vi "PicoScope5000aAWG.vi"(6 "Arbitrary Waveform Settings":T2 {"Index Mode" items=["Single", "Dual", "Quad"]}, 7 "Standard Waveform Settings":T1={"Start Frequency"=1000.0, "Stop Frequency"=1000.0, "Increment"=0.0, "Dwell Time (seconds)"=0.0} {"Stop Frequency" min=0.03 max=1000000.0; "Start Frequency" min=0.03 max=1000000.0}, 9 "General AWG Settings":T3={"Peak-to-Peak Voltage (microvolts)"=2000000, "Offset Voltage (microvolts)"=0, "Wave Type"=0, "Sweep Type"=0, "Shots"=0, "Sweeps"=0, "Trigger Type"=0, "Trigger Source"=0, "Ext. Threshold (ADC count)"=0, "White Noise/PRBS"=0} {"White Noise/PRBS" items=["Normal", "White Noise", "PRBS"]; "Trigger Source" items=["None", "Scope Trigger", "Aux. In", "Ext. In", "Software Trigger"]; "Trigger Type" items=["Rising", "Falling", "Gate High", "Gate Low"]; "Sweep Type" items=["Up", "Down", "Up-Down", "Down-Up"]; "Wave Type" items=["Sine", "Square", "Triangle", "Ramp Up", "Ramp Down", "Sinc", "Gaussian", "Half Sine", "DC", "Arbitrary"]}, 10 "Handle In":i16, 11 "error in":errorcluster) -> (0 "Trigger Source Out":u32, 1 "Arbitrary\nWaveform Graph":i16[](graph), 2 "Handle Out":i16, 3 "error out":errorcluster)   [LabVIEW 2010]
doc: "This VI can be used to control the arbitrary waveform generator. Standard waveforms can be selected or arbitrary waveform can be selected under 'Wave Type'. There are three settings clusters: general settings that apply to both arbitrary and standard waveforms, settings that apply only to standard waveforms and settings that apply only to arbitrary waveforms. It is not necessary to connect all of these clusters if only using arbitrary waveforms or only using standard waveforms are required.\n\nWhen selecting arbitrary waveform, it is necessary to specify a text file containing the wave form. This text file should have a single value on each line in the range -1 to 1. For further information on the settings, see descriptions of ps3000aSetSigGenBuiltIn and ps3000aSetSigGenArbitrary."
uses:
  ps5000a.dll
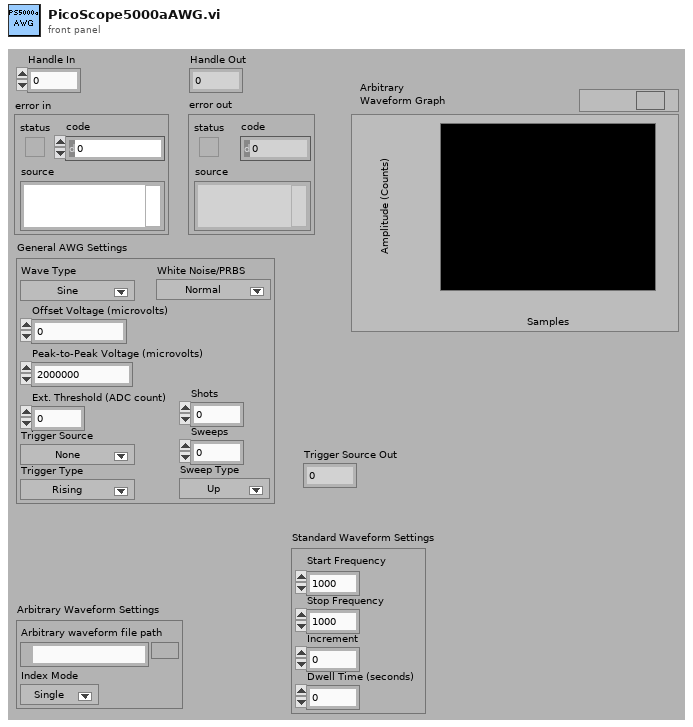
[diagram p1: front panel]
types:
  T1 = cluster{"Start Frequency":dbl, "Stop Frequency":dbl, "Increment":dbl, "Dwell Time (seconds)":dbl}
  T2 = cluster{"Arbirary waveform file path":path, "Index Mode":u32}
  T3 = cluster{"Peak-to-Peak Voltage (microvolts)":u32, "Offset Voltage (microvolts)":i32, "Wave Type":u32, "Sweep Type":u32, "Shots":u32, "Sweeps":u32, "Trigger Type":u32, "Trigger Source":u32, "Ext. Threshold (ADC count)":i16, "White Noise/PRBS":u32}
  T4 = cluster{"status":bool, "code":u32, "source":string}
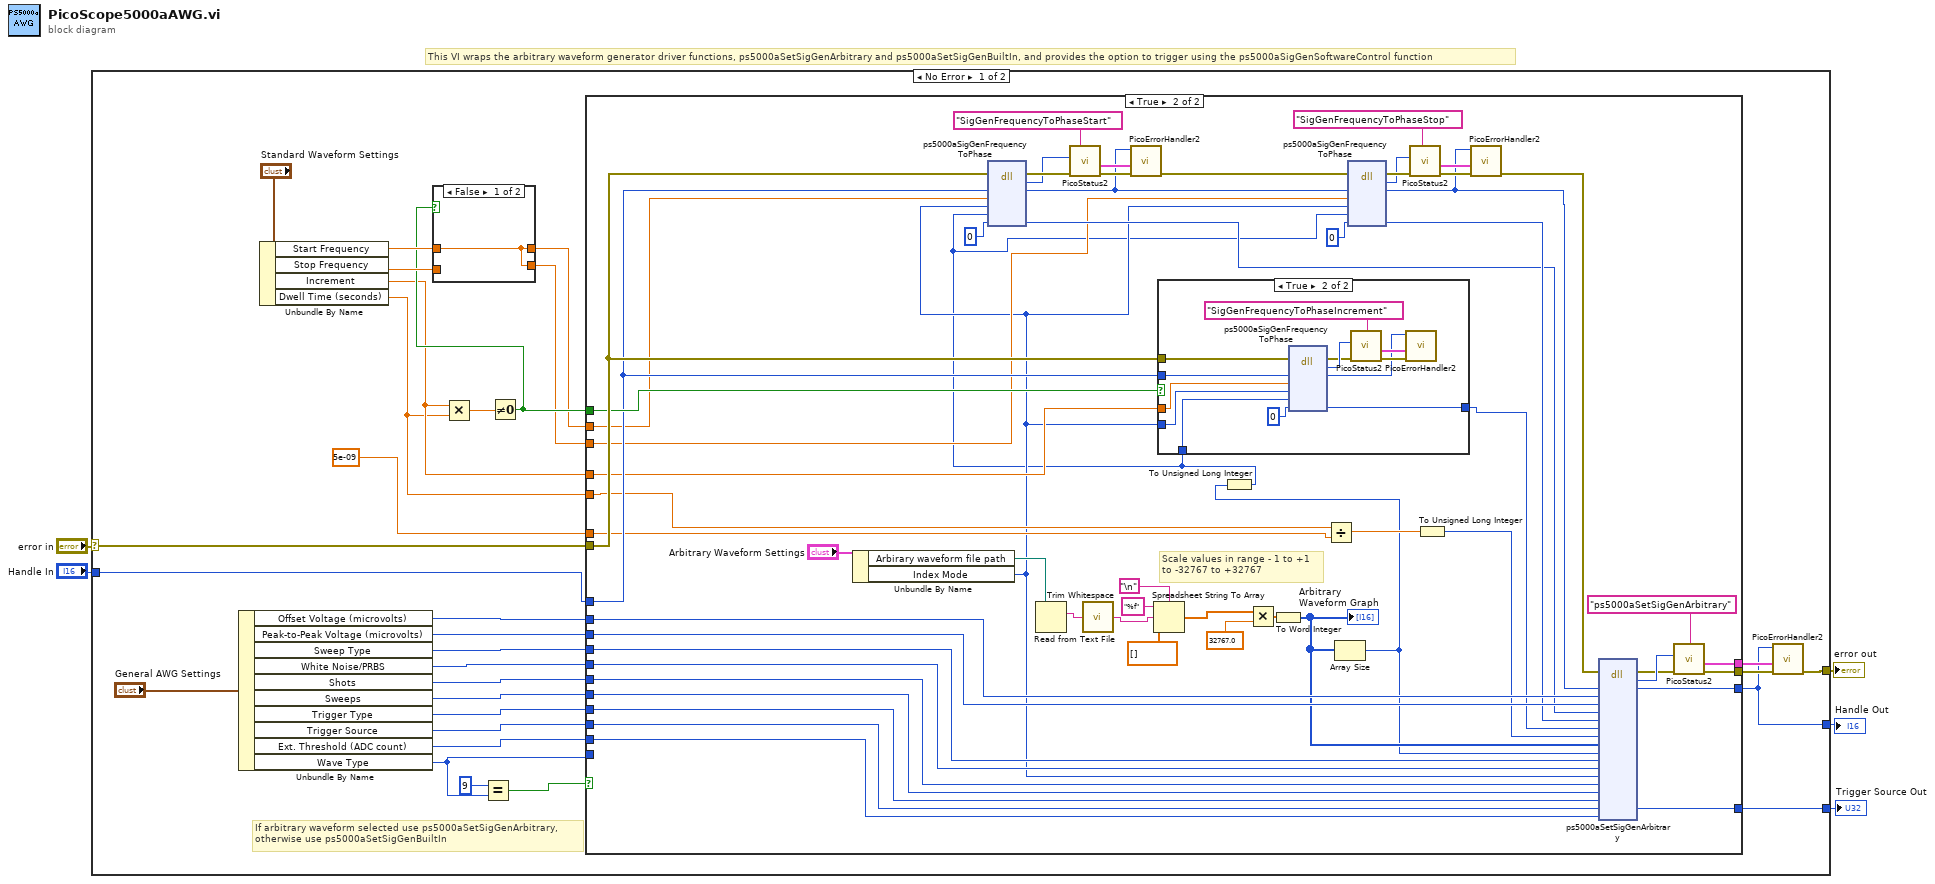
[diagram p0: block diagram]
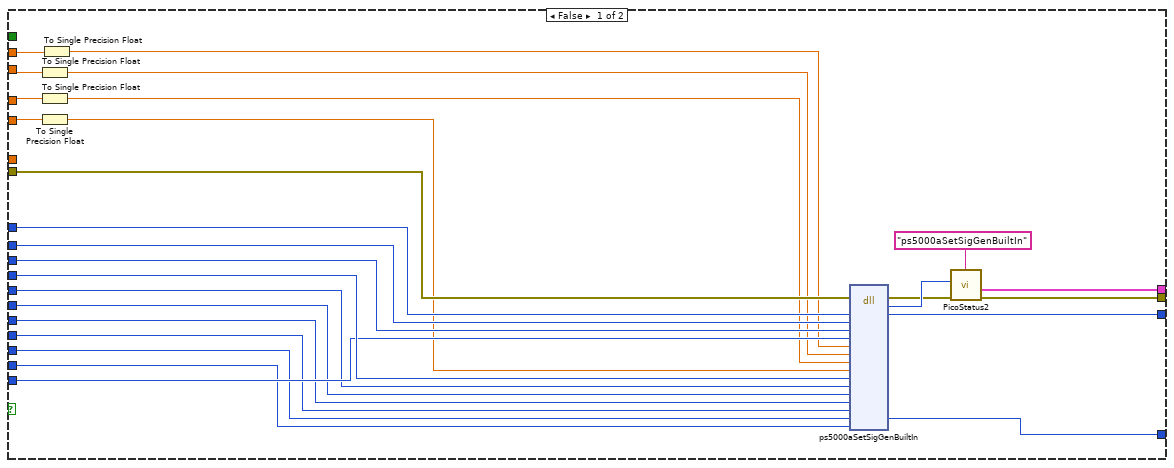
[diagram p3: hidden frame]
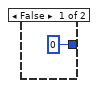
[diagram p4: hidden frame]
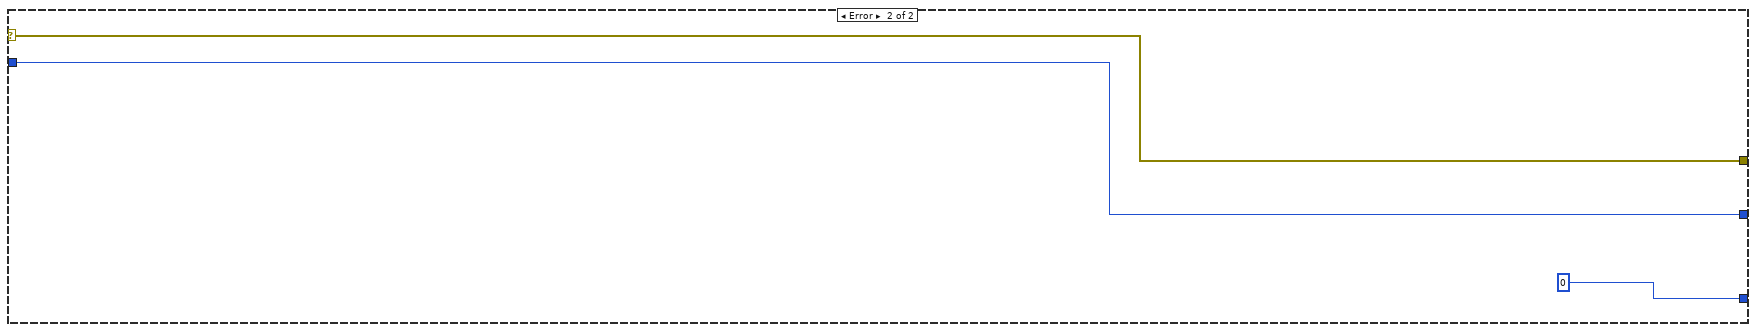
[diagram p5: hidden frame]
diagram:
  # "This VI wraps the arbitrary waveform generator driver functions, ps5000aSetSigGenArbitrary and ps5000aSetSigGenBuiltIn, and provides the option to trigger using the ps5000aSigGenSoftwareControl function"
  n1 = case shown="No Error" "error in" {
    selector: "error in" -> [w20 w141]
    tunnel: [w6 w140] -> w5
    tunnel: "Handle In" -> [w33 w140]
    tunnel: [w32 w141] -> w3
    tunnel: [w18 0] -> w1
    frame No Error {
      # "If arbitrary waveform selected use ps5000aSetSigGenArbitrary, \notherwise use ps5000aSetSigGenBuiltIn"
      n2 = Unbundle By Name("General AWG Settings") -> ("Offset Voltage (microvolts)"=w30:i32, "Peak-to-Peak Voltage (microvolts)"=w29:u32, "Sweep Type"=w28:u32, "White Noise/PRBS"=w27:u32, "Shots"=w26:u32, "Sweeps"=w25:u32, "Trigger Type"=w24:u32, "Trigger Source"=w23:u32, "Ext. Threshold (ADC count)"=w22:i16, "Wave Type"=w21:u32)
      n3 = Unbundle By Name("Standard Waveform Settings") -> ("Start Frequency"=w16:dbl, "Stop Frequency"=w15:dbl, "Increment"=w10:dbl, "Dwell Time (seconds)"=w9:dbl)
      n4 = Multiply(x=w10, y=w9) -> (x*y=w14:dbl)
      n5 = Equal?(x=u32 9, y=w21) -> (x = y?=w35:bool)
      n6 = Not Equal To 0?(x=w14) -> (x != 0?=w13:bool)
      n7 = case shown="False" w13 {
        tunnel: [w36 w38] -> w11
        tunnel: w15 -> [_ w38]
        tunnel: w16 -> [w36 w37]
        tunnel: [w36 w37] -> w12
        frame False {
        }
        frame True {
        }
      }
      n8 = case shown="True" w35 {
        tunnel: [w65 w119] -> w6
        tunnel: w33 -> [w64 w83]
        tunnel: [w62 w116] -> w19
        tunnel: w30 -> [w60 w115]
        tunnel: w29 -> [w59 w114]
        tunnel: w28 -> [w58 w113]
        tunnel: w27 -> [w48 w101]
        tunnel: w26 -> [w56 w112]
        tunnel: w25 -> [w55 w111]
        tunnel: w24 -> [w54 w110]
        tunnel: w23 -> [w53 w109]
        tunnel: w22 -> [w52 w106]
        tunnel: w21 -> [w57 _]
        tunnel: [w51 w104] -> w18
        tunnel: w20 -> [w50 w86]
        tunnel: w13 -> [_ w84]
        tunnel: w12 -> [w47 w82]
        tunnel: w11 -> [w46 w81]
        tunnel: w10 -> [w45 w78]
        tunnel: w9 -> [w44 w79]
        tunnel: 5e-09 ("y") -> [_ w80]
        tunnel: [w39 w70] -> w7
        frame False {
          n9 = To Single Precision Float(number=w46) -> (single precision float=w41:sgl)
          n10 = To Single Precision Float(number=w45) -> (single precision float=w42:sgl)
          n11 = To Single Precision Float(number=w44) -> (single precision float=w43:sgl)
          n12 = To Single Precision Float(number=w47) -> (single precision float=w40:sgl)
          n13 = dll-call lib="ps5000a.dll" fn="ps5000aSetSigGenBuiltIn" ("ps3000.dll:_ps3000_open_unit@0")(error in=w50, "handle"=w64, "offsetVoltage"=w60, "pkToPk"=w59, "waveType"=w57, "startFrequency"=w40, "stopFrequency"=w41, "increment"=w42, "dwellTime"=w43, "sweepType"=w58, "operation"=w48, "shots"=w56, "sweeps"=w55, "triggerType"=w54, "triggerSource"=w53, "extInThreshold"=w52) -> (error out=w49:errorcluster, "PICO_STATUS"=w63:u32, "handle"=w65:i16, "triggerSource"=w51:u32)  [unwired: 15 in, 1 out]
          n14 = call "PicoStatus2.vi"("PICO source"="ps5000aSetSigGenBuiltIn" ("source"), "Error in"=w49, "PICO STATUS"=w63) -> ("error out"=w62:errorcluster, "PICO_STATUS out"=w39:T4)  [unwired: 5 in]
        }
        frame True {
          # "Scale values in range - 1 to +1 \nto -32767 to +32767"
          n15 = Unbundle By Name("Arbitrary Waveform Settings") -> ("Arbirary waveform file path"=w107:path, "Index Mode"=w77:u32)
          n16 = Read from Text File(file (use dialog)=w107) -> (text=w72:string)  [unwired: 3 in, 3 out]
          n17 = call <vilib>:"Trim Whitespace.vi"("string"=w72) -> ("trimmed string"=w71:string)  [unwired: 1 in]
          n18 = Spreadsheet String To Array(delimiter (Tab)="\n", format string="%f", spreadsheet string=w71, array type (2D Dbl)=dbl[] []) -> (array=w120:dbl[])
          n19 = Multiply(x=w120, y=32767.0 ("deltaPhaseIncrement")) -> (x*y=w102:dbl[])
          n20 = To Word Integer(number=w102) -> (16bit integer=w105:i16[])
          "Arbitrary\nWaveform Graph" <- w105
          n21 = Divide(x=w79, y=w80) -> (x/y=w76:dbl)
          n22 = Array Size(array=w105) -> (size(s)=w73:i32)
          n23 = To Unsigned Long Integer(number=w73) -> (unsigned 32bit integer=w74:u32)
          n24 = dll-call lib="ps5000a.dll" fn="ps5000aSigGenFrequencyToPhase" ("ps3000.dll:_ps3000_open_unit@0")(error in=w86, "handle"=w83, "frequency"=w82, "indexMode"=w77, "bufferLength"=w74, "phase"=u32 0) -> (error out=w98:errorcluster, "PICO_STATUS"=w97:u32, "handle"=w66:i16, "phase"=w85:u32)  [unwired: 5 in, 1 out]
          n25 = call "PicoStatus2.vi"("PICO source"="SigGenFrequencyToPhaseStart" ("source"), "Error in"=w98, "PICO STATUS"=w97) -> ("error out"=w100:errorcluster, "PICO_STATUS out"=w67:T4)  [unwired: 5 in]
          n26 = call "PicoErrorHandler2.vi"("error in (no error)"=w100, "PICO_STATUS in"=w67, "handle In"=w66) -> ("error out"=w92:errorcluster)  [unwired: 8 in]
          n27 = case shown="True" w84 {
            tunnel: w86 -> [_ w134]
            tunnel: w83 -> [_ w133]
            tunnel: w78 -> [_ w132]
            tunnel: w74 -> [_ w130]
            tunnel: [u32 0 ("phase") w129] -> w87
            tunnel: w77 -> [_ w128]
            frame False {
            }
            frame True {
              n28 = dll-call lib="ps5000a.dll" fn="ps5000aSigGenFrequencyToPhase" ("ps3000.dll:_ps3000_open_unit@0")(error in=w134, "handle"=w133, "frequency"=w132, "indexMode"=w128, "bufferLength"=w130, "phase"=u32 0) -> (error out=w137:errorcluster, "PICO_STATUS"=w138:u32, "handle"=w126:i16, "phase"=w129:u32)  [unwired: 5 in, 1 out]
              n29 = call "PicoStatus2.vi"("PICO source"="SigGenFrequencyToPhaseIncrement" ("source"), "Error in"=w137, "PICO STATUS"=w138) -> ("error out"=w135:errorcluster, "PICO_STATUS out"=w127:T4)  [unwired: 5 in]
              n30 = call "PicoErrorHandler2.vi"("error in (no error)"=w135, "PICO_STATUS in"=w127, "handle In"=w126) -> ()  [unwired: 8 in, 1 out]
            }
          }
          n31 = dll-call lib="ps5000a.dll" fn="ps5000aSigGenFrequencyToPhase" ("ps3000.dll:_ps3000_open_unit@0")(error in=w92, "handle"=w66, "frequency"=w81, "indexMode"=w77, "bufferLength"=w74, "phase"=u32 0) -> (error out=w94:errorcluster, "PICO_STATUS"=w93:u32, "handle"=w68:i16, "phase"=w88:u32)  [unwired: 5 in, 1 out]
          n32 = call "PicoStatus2.vi"("PICO source"="SigGenFrequencyToPhaseStop" ("source"), "Error in"=w94, "PICO STATUS"=w93) -> ("error out"=w96:errorcluster, "PICO_STATUS out"=w69:T4)  [unwired: 5 in]
          n33 = To Unsigned Long Integer(number=w76) -> (unsigned 32bit integer=w75:u32)
          n34 = call "PicoErrorHandler2.vi"("error in (no error)"=w96, "PICO_STATUS in"=w69, "handle In"=w68) -> ("error out"=w89:errorcluster)  [unwired: 8 in]
          n35 = dll-call lib="ps5000a.dll" fn="ps5000aSetSigGenArbitrary" ("ps3000.dll:_ps3000_open_unit@0")(error in=w89, "handle"=w68, "offsetVoltage"=w115, "pkToPk"=w114, "startDeltaPhase"=w85, "stopDeltaPhase"=w88, "deltaPhaseIncrement"=w87, "dwellCount"=w75, "arbitraryWaveform"=w105, "arbitraryWaveformSize"=w73, "sweepType"=w113, "operation"=w101, "indexMode"=w77, "shots"=w112, "sweeps"=w111, "triggerType"=w110, "triggerSource"=w109, "extInThreshold"=w106) -> (error out=w103:errorcluster, "PICO_STATUS"=w118:u32, "handle"=w119:i16, "triggerSource"=w104:u32)  [unwired: 17 in, 1 out]
          n36 = call "PicoStatus2.vi"("PICO source"="ps5000aSetSigGenArbitrary" ("source"), "Error in"=w103, "PICO STATUS"=w118) -> ("error out"=w116:errorcluster, "PICO_STATUS out"=w70:T4)  [unwired: 5 in]
        }
      }
      n37 = call "PicoErrorHandler2.vi"("error in (no error)"=w19, "PICO_STATUS in"=w7, "handle In"=w6) -> ("error out"=w32:errorcluster)  [unwired: 8 in]
    }
    frame Error {
    }
  }
  "Handle Out" <- w5
  "error out" <- w3
  "Trigger Source Out" <- w1
